vi "Save Transport ITX File.vi"(8 "error in (no error)":errorcluster, 11 "Control Experiment in":refnum<class "Control Experiment.lvclass">) -> (0 "error out":errorcluster, 3 "Control Experiment out":refnum<class "Control Experiment.lvclass">)   [LabVIEW 2019, in "Control Experiment.lvclass"]
uses:
  Control Experiment.lvclass
  <userlib>/LevyLab/LV-Data/LV-Data/Typedefs/File Type--enum.ctl
  Control Experiment.lvclass/Control Experiment.ctl
  <userlib>/LevyLab/LV-Data/LV-Data/LV-Data.lvclass
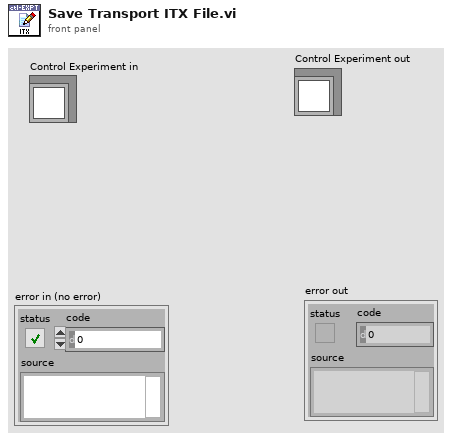
[diagram p1: front panel]
types:
  T1 = typedef "LV-Data.lvclass/File Type--enum.ctl" = enum16{"DAT", "ITX", "TDMS", "VI"}
  T2 = typedef "LV-Data.lvclass/Dictionary--cluster.ctl" = cluster{"key":string, "value":variant}
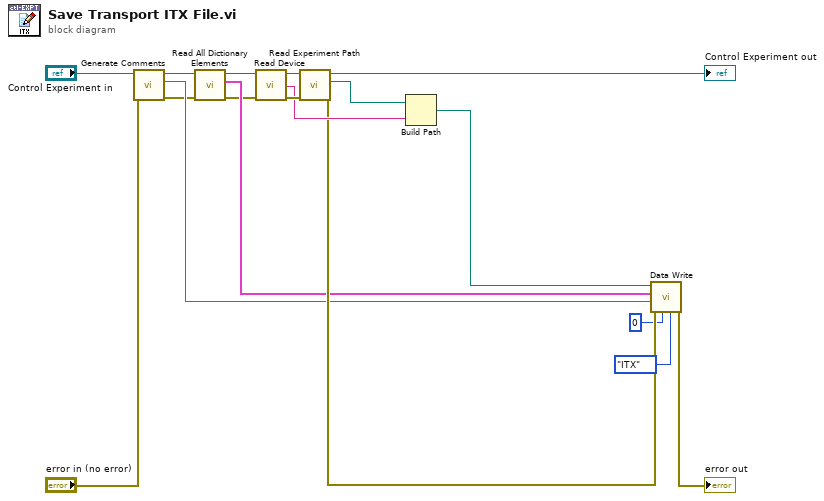
[diagram p0: block diagram]
diagram:
  n1 = call "Generate Comments.vi"("error in (no error)"="error in (no error)", "Control Experiment"="Control Experiment in") -> ("error out"=w6:errorcluster, "Comments"=w7:string, "Control Experiment out"=w5:refnum<class "Control Experiment.lvclass">)  [unwired: 6 in]
  n2 = call "Read All Dictionary Elements.vi"("error in (no error)"=w6, "Control Experiment in"=w5) -> ("error out"=w1:errorcluster, "Items"=w3:T2[], "Control Experiment out"=w4:refnum<class "Control Experiment.lvclass">)  [unwired: 7 in]
  n3 = call "Read Device.vi"("error in (no error)"=w1, "Control Experiment in"=w4) -> ("error out"=w16:errorcluster, "Device"=w11:string, "Control Experiment out"=w17:refnum<class "Control Experiment.lvclass">)  [unwired: 7 in]
  n4 = call "Read Experiment Path.vi"("error in (no error)"=w16, "Control Experiment in"=w17) -> ("error out"=w9:errorcluster, "Experiment Path"=w12:path, "Control Experiment out"=→"Control Experiment out":refnum<class "Control Experiment.lvclass">)  [unwired: 7 in]
  n5 = Build Path(base path=w12, name or relative path=w11) -> (appended path=w10:path)
  n6 = call <userlib>:"Data Write.vi"("File Type"=File_Type--enum."ITX", "Append Index"=0, "error in (no error)"=w9, "Notes"=w7, "Data (Dictionary)"=w3, "path"=w10) -> ("error out"=→"error out":errorcluster)  [unwired: 4 in, 1 out]
